vi "PCO_GetFastTimingMode.vi"(8 "error in (no error)":errorcluster {"code" format="%x"}, 11 "ph":u64) -> (0 "error out":errorcluster {"code" format="%x"}, 1 "wFastTimingMode":u16(ring) items=["OFF", "ON"], 2 "ErrorMessage":i32 format="%x", 3 "ph out":u64)   [LabVIEW 2019, in "SDK.lvlib" / "TimingControl.lvlib"]
doc: "<b>Description:</b>\nThis function returns the current fast timing mode setting of the camera.\n\nIf the camera is set to fast timing mode image timing is changed. The interframing time between two images is reduced to to 3.5 ìs despite the normal value of about 75 ìs. While running in fast timing mode image quality is reduced, which might be acceptable for special applications like PIV.\n\n<b>Supported camera type:</b>\npco.dimax\n\n<b>Descriptor dependency:</b>\ndwGeneralCapsDESC1: FAST_TIMING"
uses:
  TimingControl.lvlib
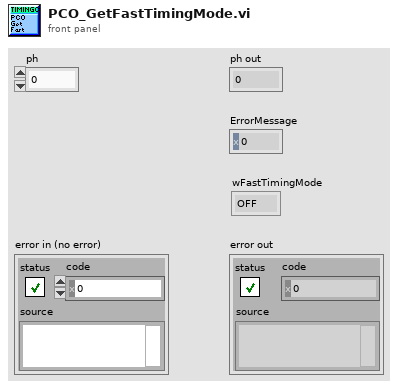
[diagram p1: front panel]
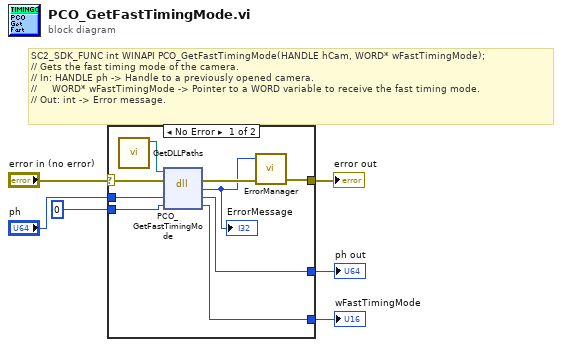
[diagram p0: block diagram]
diagram:
  # "SC2_SDK_FUNC int WINAPI PCO_GetFastTimingMode(HANDLE hCam, WORD* wFastTimingMode);\n// Gets the fast timing mode of the camera.\n// In: HANDLE ph -> Handle to a previously opened camera.\n//     WORD* wFastTimingMode -> Pointer to a WORD variable to receive the fast timing mode.\n// Out: int -> Error message."
  n1 = case shown="No Error" "error in (no error)" {
    selector: "error in (no error)" -> [w11 w18]
    tunnel: "ph" -> [w15 w17]
    tunnel: [w14 w17] -> w5
    tunnel: u16 0 ("wFastTimingMode") -> [w13 w16]
    tunnel: [w12 w16] -> w3
    tunnel: [w9 w18] -> w2
    frame No Error {
      n2 = call "GetDLLPaths.vi"() -> ("SC2_Cam_Path"=w7:path)  [unwired: 8 in, 3 out]
      n3 = dll-call lib="?" fn="PCO_GetFastTimingMode"(path in=w7, error in=w11, "ph"=w15, "wFastTimingMode"=w13) -> (error out=w10:errorcluster, "return type"=w8:i32, "ph"=w14:u64, "wFastTimingMode"=w12:u16)  [unwired: 1 in, 1 out]
      "ErrorMessage" <- w8
      n4 = call "ErrorManager.vi"("error in (no error)"=w10, "error code"=w8) -> ("error out"=w9:errorcluster)  [unwired: 2 in, 1 out]
    }
    frame Error {
    }
  }
  "ph out" <- w5
  "wFastTimingMode" <- w3
  "error out" <- w2
